vi "SSIM.vi"() -> ()   [LabVIEW 2014]
doc: "This example shows how to use the Structural Similarity Analysis tools in NI Vision. \n\nSSIM is a metric used to determine the Similarity of an Image with respect to a Reference Image. The Reference Image is assumed to be of perfect quality. SSIM uses a window based approach and uses the structural information to determine the similarity unlike the Mean Square Error which isolates the pixels from its neighbouring pixels.\n\nThere are two SSIM techniques. Fast and Normal SSIM. Fast SSIM uses faster approaches to calculate the mean and variance. Fast SSIM calculates mean by averaging pixel values in the local window whereas Normal SSIM uses a Gaussian weighting function."
uses:
  <vilib>/vision/NI_Vision_Development_Module.lvlib
panel:
  in  "Window Size":i32=7
  out "Mean Square Error":dbl
  out "Mean SSIM*":dbl
  out "MSE Map":T1(plugin-control)
  out "SSIM Map":T1(plugin-control)
  out "Test Image":T1(plugin-control)
  out "Ref Image":T1(plugin-control)
  # "* In SSIM the value 1 indicates the images are similar, the value 0 indicates the images are dissimilar."
  # "Comparison Results"
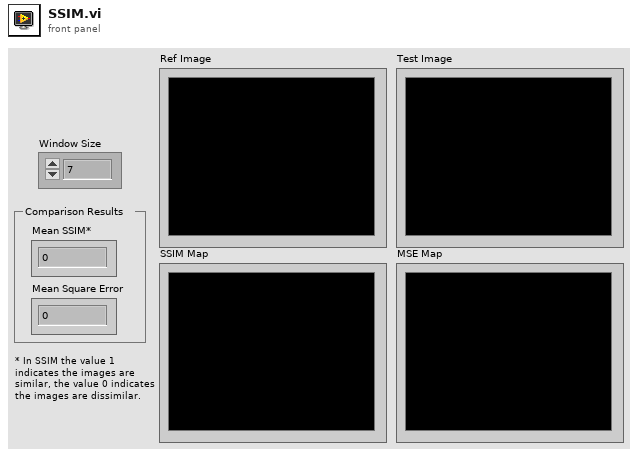
[diagram p1: front panel]
types:
  T1 = typedef "IMAQ Image.ctl" = refnum<image>
  T2 = typedef "Image Type" = u32
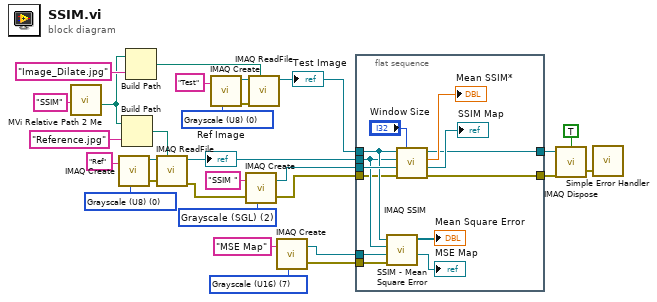
[diagram p0: block diagram]
diagram:
  w3 = T2 7 items=["Grayscale (U8)", "Grayscale (I16)", "Grayscale (SGL)", "Complex (CSG)", "RGB (U32)", "HSL (U32)", "RGB (U64)", "Grayscale (U16)"] ("Image Type")
  w19 = T2 2 items=["Grayscale (U8)", "Grayscale (I16)", "Grayscale (SGL)", "Complex (CSG)", "RGB (U32)", "HSL (U32)", "RGB (U64)"] ("Image Type")
  w23 = T2 0 items=["Grayscale (U8)", "Grayscale (I16)", "Grayscale (SGL)", "Complex (CSG)", "RGB (U32)", "HSL (U32)", "RGB (U64)"] ("Image Type")
  w24 = T2 0 items=["Grayscale (U8)", "Grayscale (I16)", "Grayscale (SGL)", "Complex (CSG)", "RGB (U32)", "HSL (U32)", "RGB (U64)"] ("Image Type")
  n1 = call "MVi Relative Path 2 Me.vi"("Relative Path"="SSIM" ("name or relative path")) -> ("Appended Dir"=w7:path)  [unwired: 5 in, 1 out]
  n2 = call "IMAQ Create"("Image Name"="Ref", "Image Type"=w23) -> ("New Image"=w22:T1, "error out"=w21:errorcluster)  [unwired: 2 in, 1 out]
  n3 = Build Path(base path=w7, name or relative path="Reference.jpg") -> (appended path=w14:path)
  n4 = Build Path(base path=w7, name or relative path="Image_Dilate.jpg") -> (appended path=w13:path)
  n5 = call "IMAQ ReadFile"("File Path"=w14, "error in (no error)"=w21, "Image"=w22) -> ("error out"=w9:errorcluster, "Image Out"=w27:T1)  [unwired: 2 in, 5 out]
  "Ref Image" <- w27
  n6 = call "IMAQ Create"("Image Name"="Test", "Image Type"=w24) -> ("New Image"=w17:T1, "error out"=w16:errorcluster)  [unwired: 2 in, 1 out]
  n7 = call "IMAQ Create"("Image Name"="SSIM ", "Image Type"=w19, "error in (no error)"=w9) -> ("New Image"=w29:T1, "error out"=w8:errorcluster)  [unwired: 1 in, 1 out]
  n8 = call "IMAQ ReadFile"("File Path"=w13, "error in (no error)"=w16, "Image"=w17) -> ("Image Out"=w28:T1)  [unwired: 2 in, 6 out]
  "Test Image" <- w28
  n9 = call "IMAQ Create"("Image Name"="MSE Map", "Image Type"=w3) -> ("New Image"=w5:T1, "error out"=w2:errorcluster)  [unwired: 2 in, 1 out]
  n10 = flat-sequence {
    tunnel: w29 -> [w42]
    tunnel: w28 -> [w41]
    tunnel: w27 -> [w40]
    tunnel: [w36] -> w11
    tunnel: w8 -> [w35]
    tunnel: [w34] -> w6
    tunnel: w5 -> [w33]
    tunnel: w2 -> [w30]
    frame #0 {
      n11 = call "SSIM - Mean Square Error.vi"("error in"=w30, "MSE Map"=w33, "Reference Image"=w40, "Test Image"=w41) -> ("MSE Map Out"=→"MSE Map":T1, "Mean Square Error"=→"Mean Square Error":dbl)  [unwired: 6 out]
      n12 = call-poly "IMAQ SSIM"("Window Size"="Window Size", "error in (no error)"=w35, "SSIM Image In"=w42, "Reference Image"=w40, "Test Image"=w41) -> ("error out"=w36:errorcluster, "SSIM Image Out"=→"SSIM Map":T1, "Mean SSIM"=→"Mean SSIM*":dbl, "Test Image Out (dup)"=w34:T1)  [unwired: 3 out]
    }
  }
  n13 = call "IMAQ Dispose"("All Images? (No)"=TRUE, "Image"=w6, "error in (no error)"=w11) -> ("error out"=w1:errorcluster)  [unwired: 3 out]
  n14 = call <vilib>:"Simple Error Handler.vi"("error in (no error)"=w1) -> ()  [unwired: 4 in, 5 out]
